vi "Save File Check and Fix Summary File.vi"(7 "LV Program":T1=enum."DOE Stand", 8 "error in (no error)":errorcluster, 11 "file path (dialog if empty)":path) -> (0 "error out":errorcluster, 3 "Summary Path":path)   [LabVIEW 2016]
uses:
  File Setup (Public)/Type Definition/Save File DOE LabView Program.ctl
  <vilib>/Utility/file.llb/Read From Spreadsheet File (string).vi
  <vilib>/Utility/file.llb/Write To Spreadsheet File (string).vi
  Save File.lvlib
  File Setup.lvlib
panel:
  out "output array":string[][](array[string])
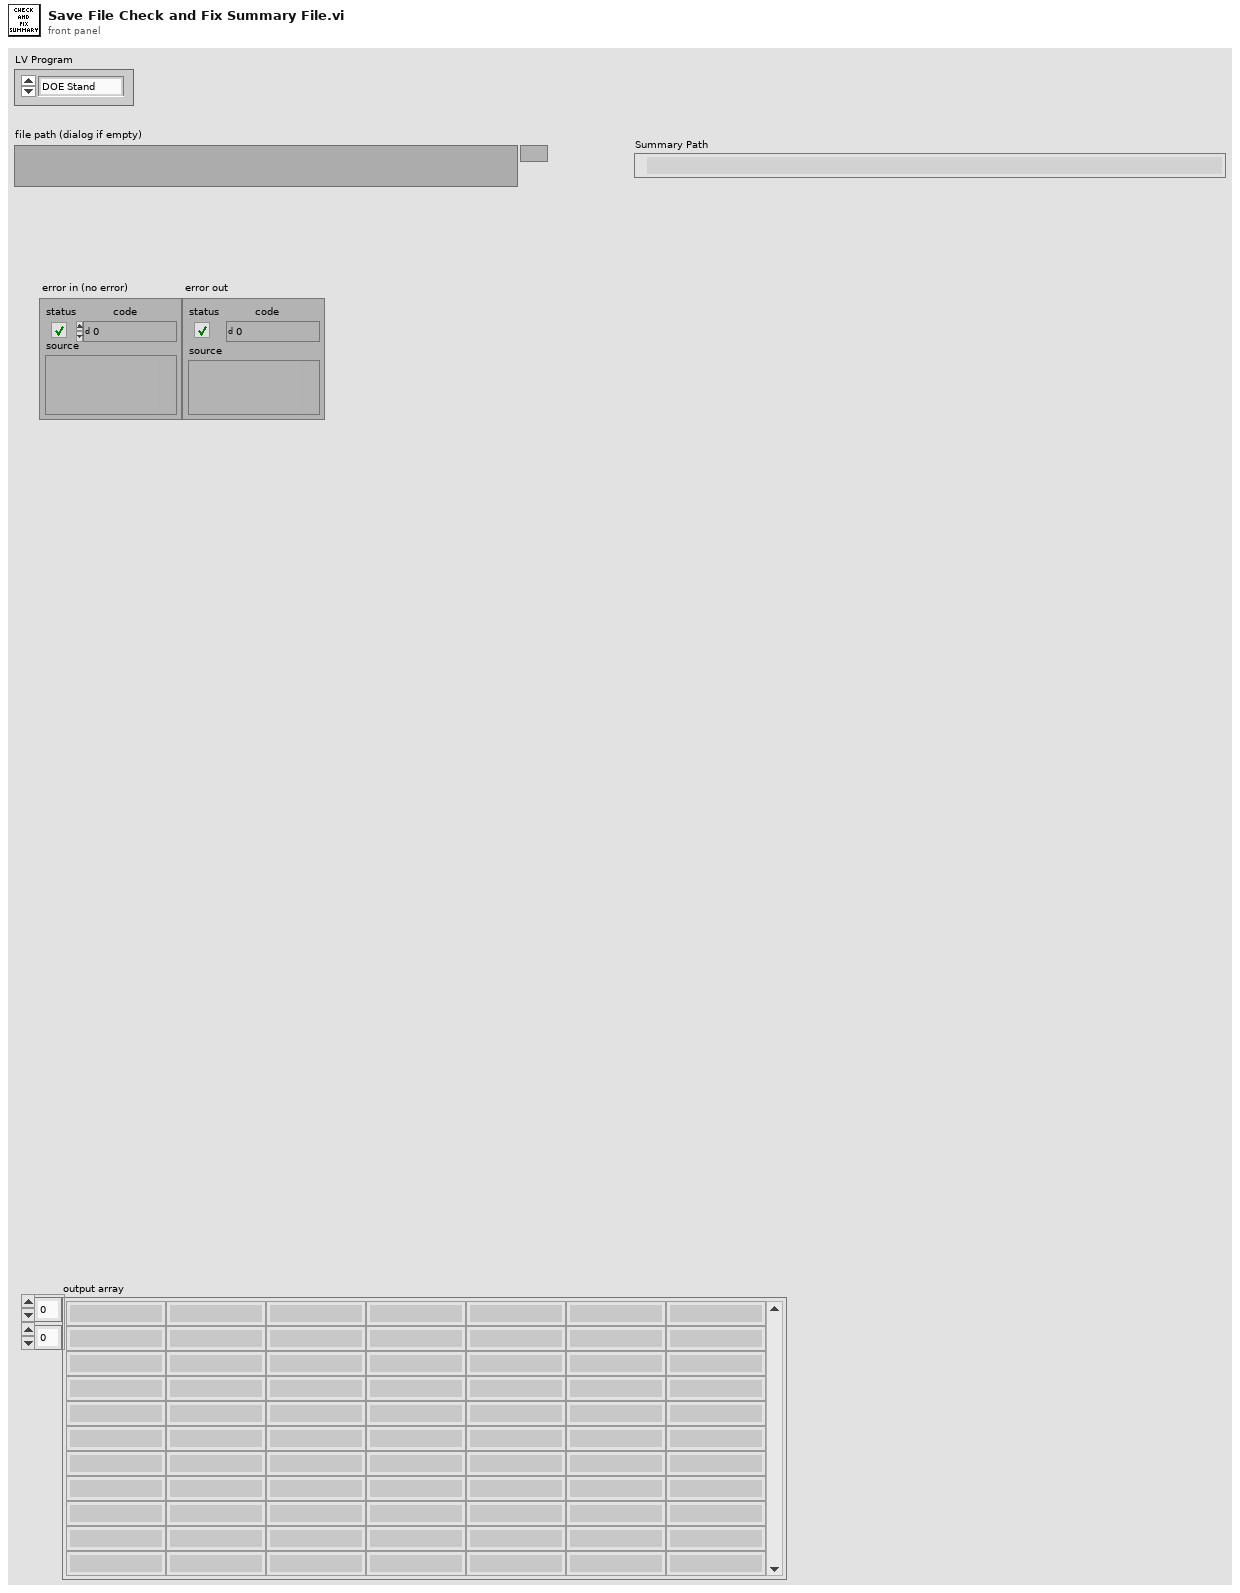
[diagram p1: front panel]
types:
  T1 = typedef "File Setup.lvlib/Save File DOE LabView Program.ctl" = enum16{"No Name Found", "DOE Stand", "Dishwasher Kitchen", "Portable Stand", "HEWH", "Dryer", "Dryer WILT", "HCC", "PRAT", "HEWH RLT", "Refrigeration"}
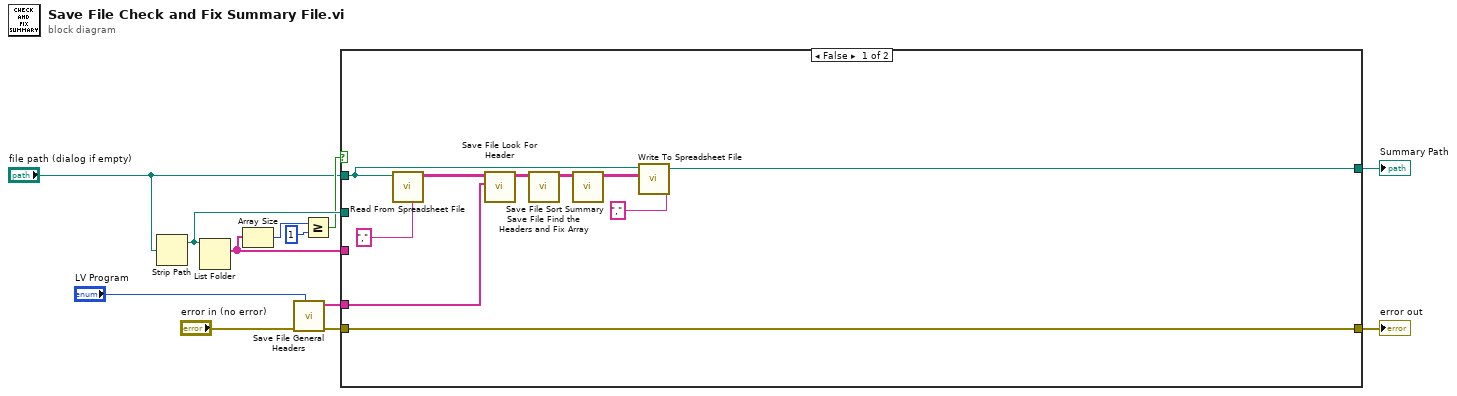
[diagram p0: block diagram]
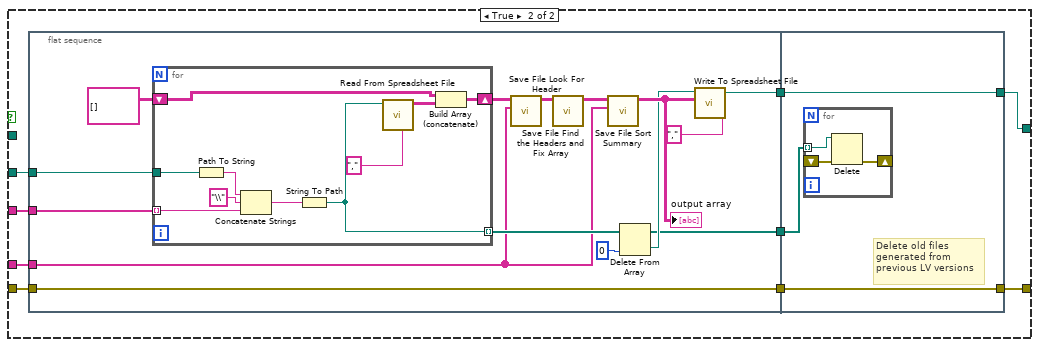
[diagram p2: hidden frame]
diagram:
  n1 = Strip Path(path="file path (dialog if empty)") -> (stripped path=w9:path)  [unwired: 1 out]
  n2 = List Folder(path=w9) -> (filenames=w10:string[])  [unwired: 3 in, 3 out]
  n3 = Array Size(array=w10) -> (size(s)=w12:i32)
  n4 = call "Save File General Headers.vi"("LV Program"="LV Program", "Error In"="error in (no error)") -> ("Error Out"=w3:errorcluster, "Summary Header"=w4:string[])  [unwired: 6 in, 2 out]
  n5 = Greater Or Equal?(x=w12, y=1) -> (x >= y?=w8:bool)
  n6 = case shown="False" w8 {
    tunnel: w10 -> [_ w31]
    tunnel: w9 -> [_ w30]
    tunnel: w4 -> [w20 w28]
    tunnel: "file path (dialog if empty)" -> [w17 _]
    tunnel: [w14 w26] -> w6
    tunnel: w3 -> [w13 w25]
    tunnel: [w13 w23] -> w5
    frame False {
      n7 = call-poly <vilib>:"Read From Spreadsheet File.vi"("delimiter (\\t)"="," ("delimiter (\\t)"), "file path (dialog if empty)"=w17) -> ("all rows"=w18:string[][])  [unwired: 5 in, 4 out]
      n8 = call "Save File Look For Header.vi"("Summary Header"=w20, "Full Data IN"=w18) -> ("Data Out"=w21:string[][])  [unwired: 8 in, 1 out]
      n9 = call "Save File Find the Headers and Fix Array.vi"("Input"=w21) -> ("Output"=w22:string[][])  [unwired: 9 in, 1 out]
      n10 = call "Save File Sort Summary.vi"("Input"=w22) -> ("Output"=w16:string[][])  [unwired: 8 in, 2 out]
      n11 = call-poly <vilib>:"Write To Spreadsheet File.vi"("delimiter (\\t)"="," ("delimiter (\\t)"), "2D data"=w16, "file path (dialog if empty)"=w17) -> ("new file path (Not A Path if cancelled)"=w14:path)  [unwired: 5 in]
    }
    frame True {
      n12 = flat-sequence {
        tunnel: w31 -> [w46]
        tunnel: w30 -> [w45]
        tunnel: [w35] -> w29
        tunnel: w28 -> [w34]
        tunnel: [w33] -> w27
        tunnel: w25 -> [w32]
        tunnel: [w32] -> w24
        tunnel: w29 -> [w59]
        tunnel: w27 -> [w58]
        tunnel: [w58] -> w26
        tunnel: w24 -> [w57]
        tunnel: [w57] -> w23
        frame #0 {
          n13 = for {
            tunnel: w46 -> [w54] mode=indexing
            tunnel: w45 -> [w56]
            shift-right: [w49] -> w44
            shift-left: string[][] [] -> [w50]
            tunnel: [w47] -> w38 mode=indexing
            n14 = Path To String(path=w56) -> (string=w55:string)
            n15 = Concatenate Strings(w55, "\\" ("string"), w54) -> (w52:string)
            n16 = String To Path(string=w52) -> (path=w47:path)
            n17 = call-poly <vilib>:"Read From Spreadsheet File.vi"("delimiter (\\t)"="," ("delimiter (\\t)"), "file path (dialog if empty)"=w47) -> ("all rows"=w48:string[][])  [unwired: 5 in, 4 out]
            n18 = Build Array (concatenate)(w50, w48) -> (w49:string[][])
          }
          n19 = call "Save File Look For Header.vi"("Summary Header"=w34, "Full Data IN"=w44) -> ("Data Out"=w43:string[][])  [unwired: 8 in, 1 out]
          n20 = call "Save File Find the Headers and Fix Array.vi"("Input"=w43) -> ("Output"=w42:string[][])  [unwired: 9 in, 1 out]
          n21 = call "Save File Sort Summary.vi"("Summary Header"=w34, "Input"=w42) -> ("Output"=w41:string[][])  [unwired: 7 in, 2 out]
          "output array" <- w41
          n22 = Delete From Array(array=w38, index=0) -> (deleted portion=w36:path, array with subset deleted=w35:path[])  [unwired: 1 in]
          n23 = call-poly <vilib>:"Write To Spreadsheet File.vi"("delimiter (\\t)"="," ("delimiter (\\t)"), "2D data"=w41, "file path (dialog if empty)"=w36) -> ("new file path (Not A Path if cancelled)"=w33:path)  [unwired: 5 in]
        }
        frame #1 {
          # "Delete old files\ngenerated from\nprevious LV versions"
          n24 = for {
            tunnel: w59 -> [w62] mode=indexing
            shift-right: [w61] -> _
            shift-left: _ -> [w60]
            n25 = Delete(path (use dialog)=w62, error in=w60) -> (error out=w61:errorcluster)  [unwired: 3 in, 2 out]
          }
        }
      }
    }
  }
  "error out" <- w5
  "Summary Path" <- w6
